vi "Get Tree Menu Data.vi"(4 "Error In":errorcluster, 7 "Menu Context":T1) -> (0 "Error Out":errorcluster, 3 "Array":T2(array[cluster]))   [LabVIEW 2020, in "Config Data.lvlib" / "Config Data.lvclass"]
uses:
  Config Data.lvclass
  Config Data.lvclass/Config Data.ctl
  typedefs/Menu Context Selections.ctl
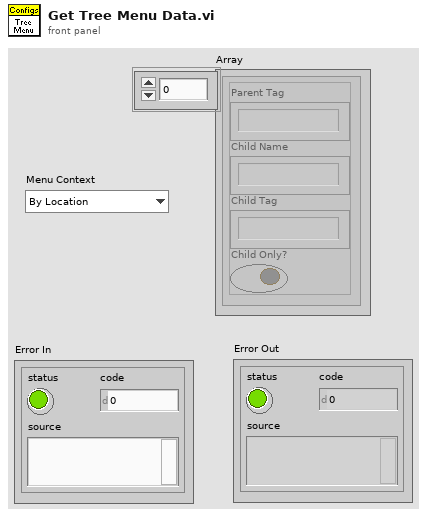
[diagram p1: front panel]
types:
  T1 = typedef "Config Data.lvlib/Config Data.lvclass/Menu Context Selections.ctl" = enum16{"By Location", "By Function"}
  T2 = cluster{"Parent Tag":string, "Child Name":string, "Child Tag":string, "Child Only?":bool}[]
  T3 = typedef "Config Data.lvlib/Config Data.lvclass/Tree Menu Entry.ctl" = cluster{"ID":i32, "Item Name":string, "Parent ID":i32, "Child Only?":bool}
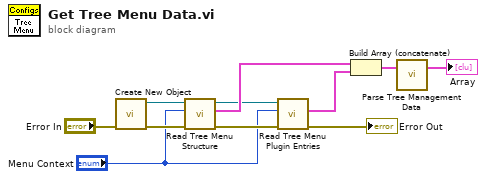
[diagram p0: block diagram]
diagram:
  n1 = call "Create New Object.vi"("Error In"="Error In") -> ("Error Out"=w11:errorcluster, "Config Data"=w10:refnum<class "Config Data.lvclass">)  [unwired: 5 in]
  n2 = call-dynamic "Read Tree Menu Structure.vi"("Error In"=w11, "Menu Context"="Menu Context", "Config Data in"=w10) -> ("Error Out"=w6:errorcluster, "Tree Menu Structure"=w9:T3[], "Config Data out"=w7:refnum<class "Config Data.lvclass">)  [unwired: 2 in]
  n3 = call-dynamic "Read Tree Menu Plugin Entries.vi"("Error In"=w6, "Menu Context"="Menu Context", "Config Data in"=w7) -> ("Error Out"=→"Error Out":errorcluster, "Tree Menu Plugin Entries"=w4:T3[])  [unwired: 2 in, 1 out]
  n4 = Build Array (concatenate)(w9, w4) -> (w3:T3[])
  n5 = call "Parse Tree Management Data.vi"("Tree Menu Data"=w3) -> ("Array"=→"Array":T2)  [unwired: 2 in]
